vi "SetPathToCheck.vi"(8 "error in (no error)":errorcluster, 9 "Path to check":path, 11 "CGrapherDGML in":refnum<class "CGrapherDGML.lvclass">) -> (0 "error out":errorcluster, 3 "CGrapherDGML out":refnum<class "CGrapherDGML.lvclass">)   [LabVIEW 2020, in "DefaultExtensions.lvlib" / "CGrapherDGML.lvclass"]
uses:
  CGrapherDGML.lvclass
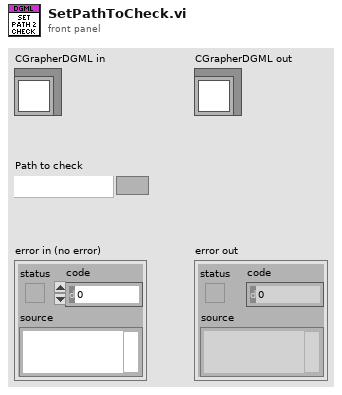
[diagram p1: front panel]
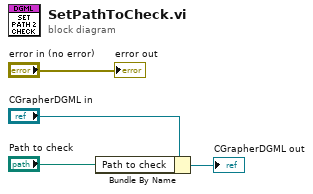
[diagram p0: block diagram]
diagram:
  n1 = Bundle By Name(cluster="CGrapherDGML in", "Path to check"="Path to check") -> (→"CGrapherDGML out":refnum<class "CGrapherDGML.lvclass">)
  "error out" <- "error in (no error)"
